vi "Demo Sensor Read.vi"(0 "VISA resource name":refnum<visa-resource-name>="COM1", 1 "baud rate":u32=9600, 2 "data bits":u16=8 min=5 max=8 step=1, 3 "parity":u16(ring) items=["None", "Odd", "Even", "Mark", "Space"], 4 "stop bits":u16(ring)=10 items=["1.0"=10, "1.5"=15, "2.0"=20], 7 "flow control":u16(ring) items=["None"=0, "XON/XOFF"=1, "RTS/CTS"=2, "DTR/DSR"=4]) -> ()   [LabVIEW 2012]
doc: "The Basic Serial Read and Write example performs a Serial Port Read, a Serial Port Write, or a combination of these actions. The user selects the actions (read or write) on the front panel. If both are selected, the VI will write the data first, read data, and then close the VISA session that is opened to the port. This VI will wait until the specified number of bytes is received at the port. Only the number of bytes specified will be read.\n\nINSTRUCTIONS:\n1) Select the serial resource and configuration parameters (baud rate, data bits, parity, stop bits, flow control).\n2) Select the operations to be performed. \n3) Connect the serial port to your device. If no device is available, perform a loopback test by doing one of the following. Short pins 2 and 3 on a RS-232 cable or short pin 4 to pin 8 and pin 5 to pin 9 on a RS-485/422 cable. \n4) Run the VI to see the data read. (The \"read string\" will match the \"string to write\" if a loopback test was performed.)\n\nNote: The parameters set for the serial port must match the parameters of the connected instrument or device. In this example, the bytes to read parameter specifies the number of bytes that the serial port reads. If there were more bytes at the port than the number specified in bytes to read, those bytes would not be read. Also, if you specify to read more bytes than the number of bytes actually read, you might receive a timeout error message.\n\nOn the block diagram, the Configure Serial Port VI sets the configuration parameters. The front panel displays the controls used to configure the basic parameters, such as baud rate, data bits, and parity. Constants configure the other parameters the user probably does not need set. After the VISA Configure Serial Port VI opens the VISA session and configures the port, the VI passes the VISA resource name to other VIs that perform operations on that VISA resource. The VISA Write function sends a command to the serial device and the VISA Read function returns data based on the command. The VISA Close function then closes the reference to the serial device. It is important to close the reference; otherwise communication through with that port through protocols other than VISA might not be possible."
uses:
  <vilib>/Instr/_visa.llb/VISA Configure Serial Port (Instr).vi
panel:
  out "Humidity":ext(graph)
  out "Temperature":ext(graph)
  out "Pressure":ext(graph)
  out "Boolean array":bool[](array[boolean])
  out "element":u8
  out "Magnetometer":cluster{ext, ext, ext}(graph)
  out "Gyro":cluster{ext, ext, ext}(graph)
  out "Accelerometer":cluster{ext, ext, ext}(graph)
  in  "stop":bool
  out "Raw Packet data (hex)":u8[](array[numeric]) format="%x"
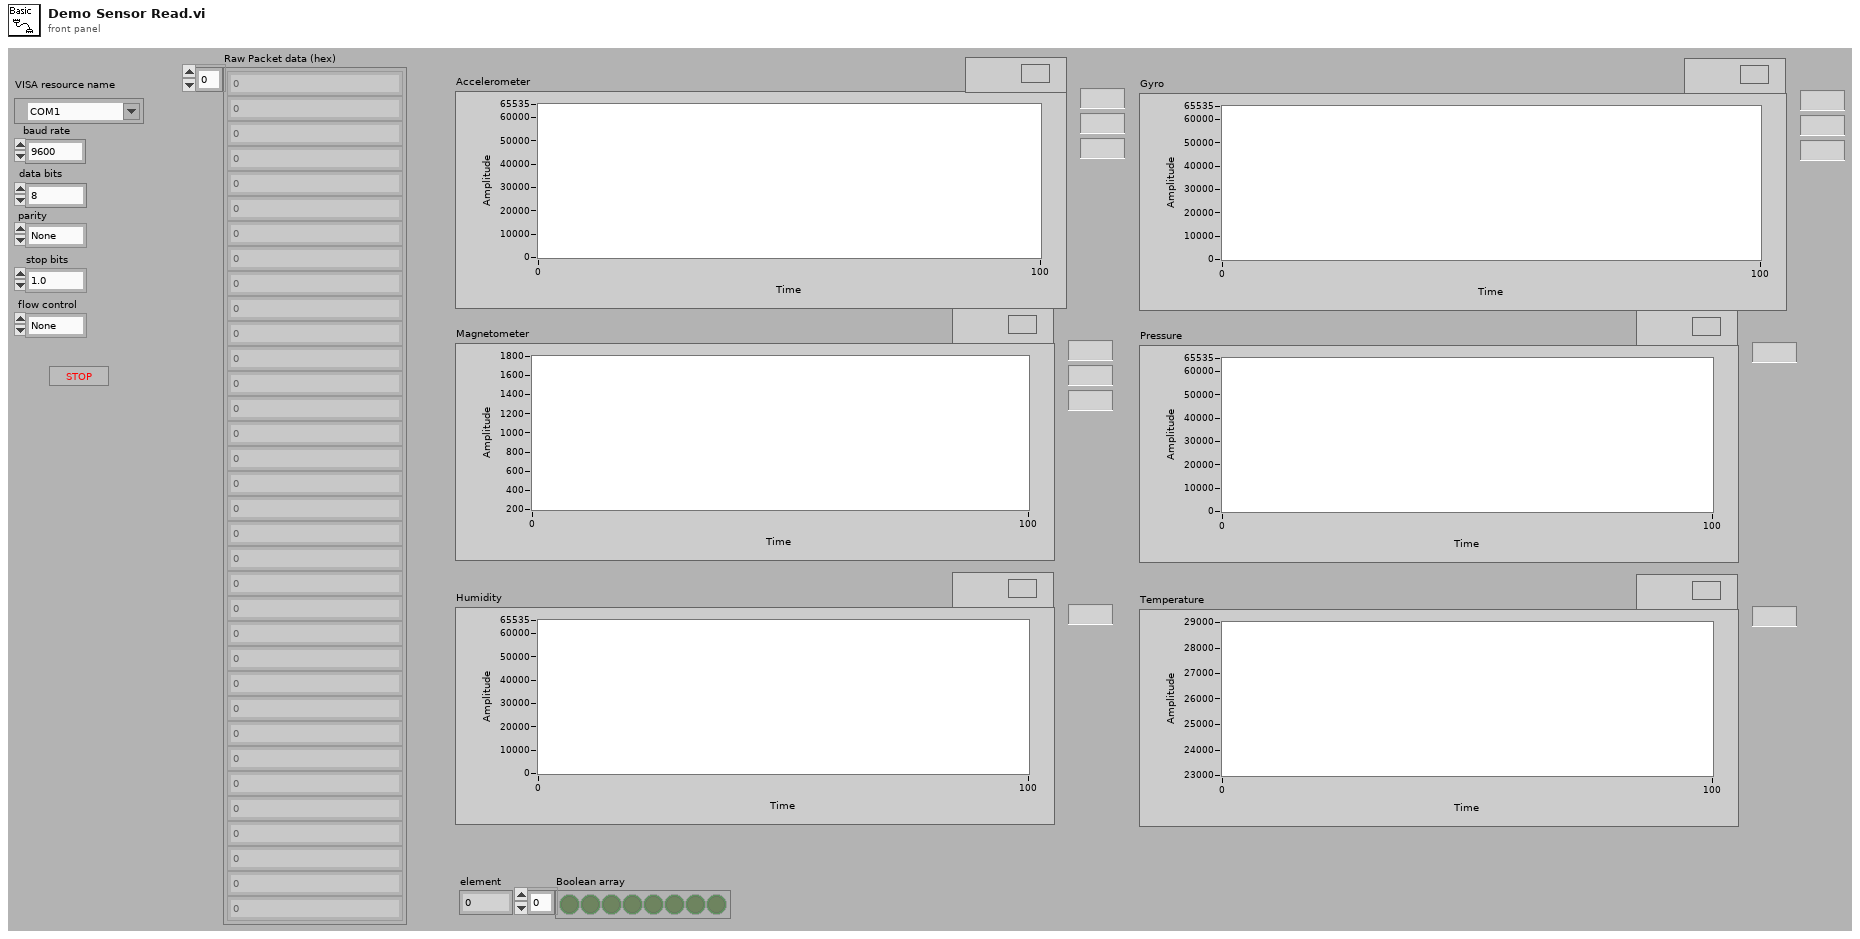
[diagram p1: front panel]
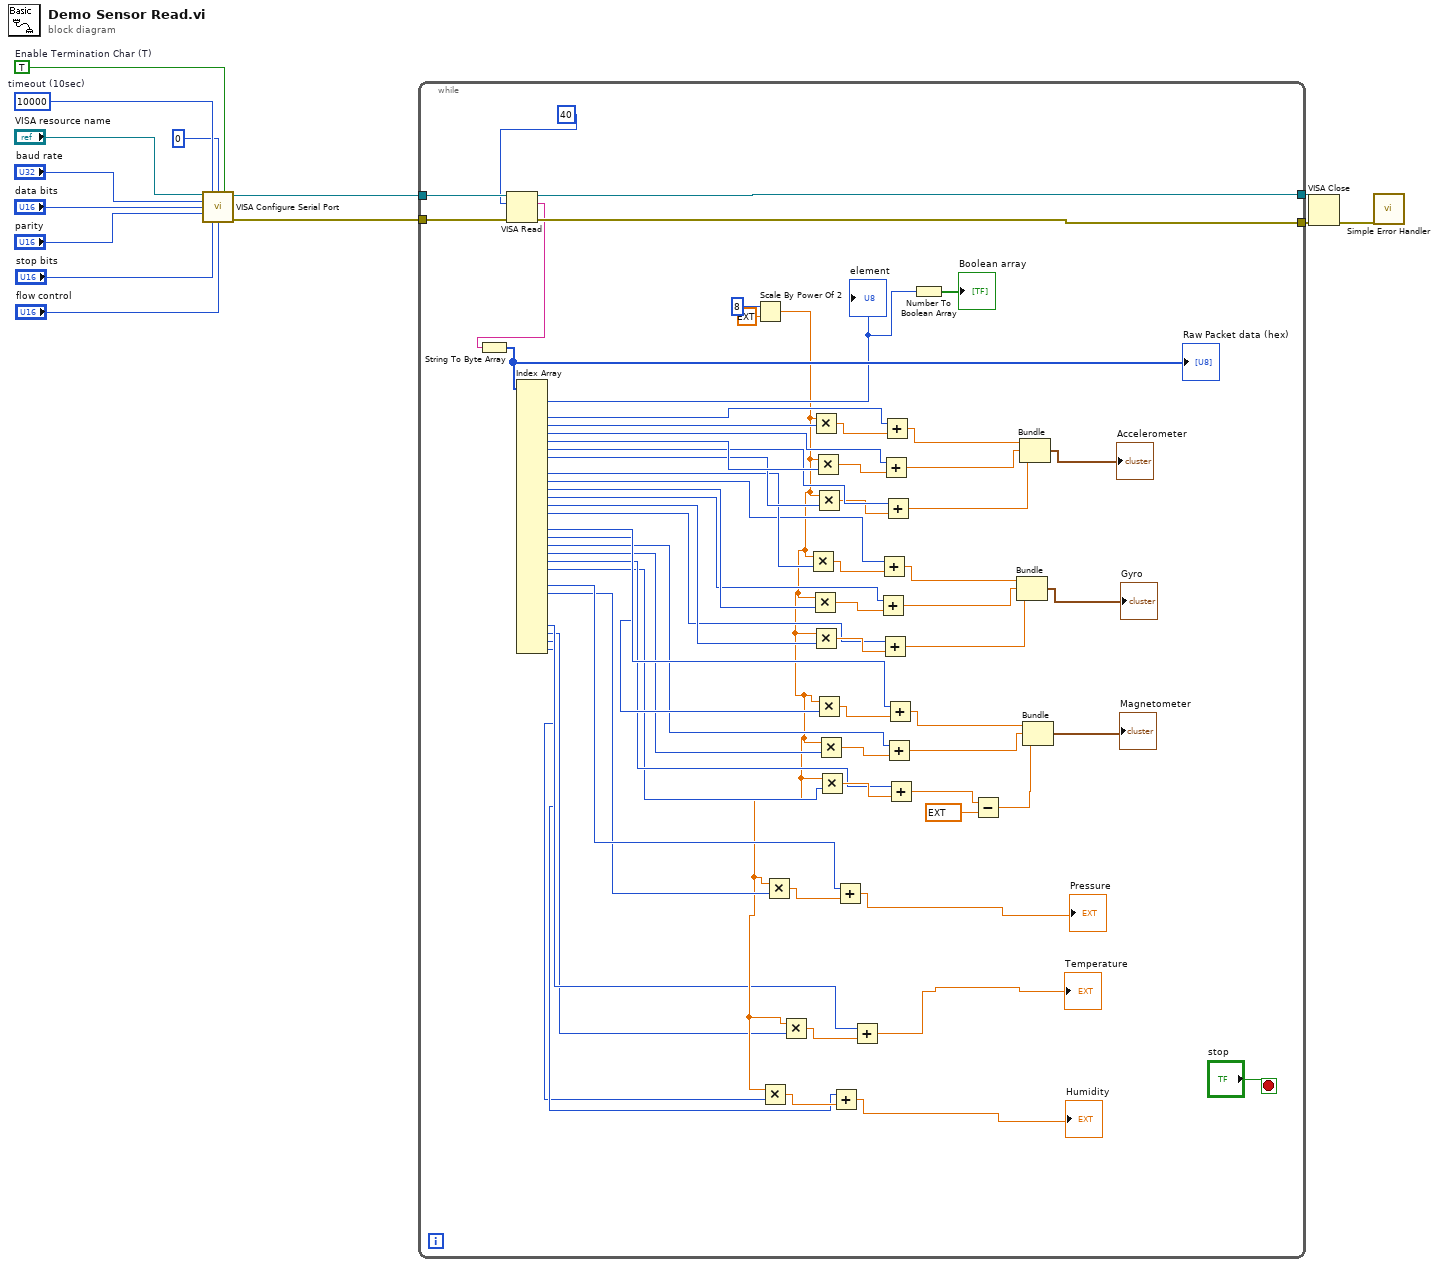
[diagram p0: block diagram]
diagram:
  w7 = TRUE  # Enable Termination Char (T)
  w8 = u32 10000  # timeout (10sec)
  n1 = call-poly "VISA Configure Serial Port"("VISA resource name"="VISA resource name", "timeout (10sec)"=w8, "termination char\n(0xA = '\\n' = LF)"=u8 0 ("termination char\n(0xA = '\\n' = LF)"), "Enable Termination\nChar (T)"=w7, "baud rate (9600)"="baud rate", "data bits (8)"="data bits", "parity (0:none)"="parity", "stop bits (10: 1 bit)"="stop bits", "flow control (0:none)"="flow control") -> ("VISA resource name out"=w3:refnum<visa-resource-name>, "error out"=w2:errorcluster)  [unwired: 5 in]
  n2 = while {
    tunnel: [w80] -> w12
    tunnel: [w79] -> w11
    tunnel: w3 -> [w78]
    tunnel: w2 -> [w77]
    stop <- "stop" stop-if-true
    n3 = VISA Read(VISA resource name=w78, byte count=40, error in (no error)=w77) -> (VISA resource name out=w79:refnum<visa-resource-name>, read buffer=w76:string, error out=w80:errorcluster)  [unwired: 1 out]
    n4 = String To Byte Array(string=w76) -> (unsigned byte array=w62:u8[])
    "Raw Packet data (hex)" <- w62
    n5 = Index Array(array=w62) -> (element #1=w61:u8, element #3=w70:u8, element #4=w73:u8, element #5=w68:u8, element #6=w72:u8, element #7=w66:u8, element #8=w71:u8, element #10=w48:u8, element #11=w45:u8, element #12=w47:u8, element #13=w44:u8, element #14=w46:u8, element #15=w43:u8, element #17=w36:u8, element #18=w35:u8, element #19=w34:u8, element #20=w33:u8, element #21=w32:u8, element #22=w31:u8, element #24=w28:u8, element #25=w27:u8, element #29=w22:u8, element #30=w21:u8, element #31=w20:u8, element #32=w19:u8)  [unwired: 32 in, 7 out]
    "element" <- w61
    n6 = Scale By Power Of 2(n=i16 8, x=ext 1.0) -> (x*2^n=w23:ext)
    n7 = Multiply(x=w23, y=w19) -> (x*y=w26:ext)
    n8 = Multiply(x=w23, y=w27) -> (x*y=w30:ext)
    n9 = Multiply(x=w23, y=w21) -> (x*y=w24:ext)
    n10 = Multiply(x=w23, y=w48) -> (x*y=w55:ext)
    n11 = Multiply(x=w23, y=w47) -> (x*y=w54:ext)
    n12 = Multiply(x=w23, y=w73) -> (x*y=w69:ext)
    n13 = Multiply(x=w23, y=w46) -> (x*y=w53:ext)
    n14 = Multiply(x=w23, y=w72) -> (x*y=w67:ext)
    n15 = Multiply(x=w23, y=w71) -> (x*y=w65:ext)
    n16 = Multiply(x=w23, y=w35) -> (x*y=w42:ext)
    n17 = Multiply(x=w23, y=w33) -> (x*y=w41:ext)
    n18 = Multiply(x=w23, y=w31) -> (x*y=w40:ext)
    n19 = Add(x=w20, y=w26) -> (x+y=→"Humidity":ext)
    n20 = Add(x=w28, y=w30) -> (x+y=→"Pressure":ext)
    n21 = Add(x=w22, y=w24) -> (x+y=→"Temperature":ext)
    n22 = Add(x=w44, y=w54) -> (x+y=w51:ext)
    n23 = Add(x=w45, y=w55) -> (x+y=w52:ext)
    n24 = Add(x=w43, y=w53) -> (x+y=w50:ext)
    n25 = Add(x=w68, y=w67) -> (x+y=w58:ext)
    n26 = Add(x=w70, y=w69) -> (x+y=w59:ext)
    n27 = Add(x=w66, y=w65) -> (x+y=w57:ext)
    n28 = Add(x=w34, y=w41) -> (x+y=w38:ext)
    n29 = Add(x=w36, y=w42) -> (x+y=w39:ext)
    n30 = Add(x=w32, y=w40) -> (x+y=w16:ext)
    n31 = Number To Boolean Array(number=w61) -> (Boolean array=→"Boolean array":bool[])
    n32 = Subtract(x=w16, y=ext 50000.0) -> (x-y=w17:ext)
    n33 = Bundle(w52, w51, w50) -> (→"Gyro":cluster{ext, ext, ext})  [unwired: 1 in]
    n34 = Bundle(w59, w58, w57) -> (→"Accelerometer":cluster{ext, ext, ext})  [unwired: 1 in]
    n35 = Bundle(w39, w38, w17) -> (→"Magnetometer":cluster{ext, ext, ext})  [unwired: 1 in]
  }
  n36 = VISA Close(VISA resource name=w11, error in (no error)=w12) -> (error out=w10:errorcluster)
  n37 = call <vilib>:"Simple Error Handler.vi"("error in (no error)"=w10) -> ()  [unwired: 4 in, 5 out]
